vi "User Input block.vi"(7 "action":T1, 8 "error in":errorcluster, 10 "Pause!":bool) -> (0 "error out":errorcluster, 2 "Pause?":bool)   [LabVIEW 2018]
uses:
  type defines/Pause action.ctl
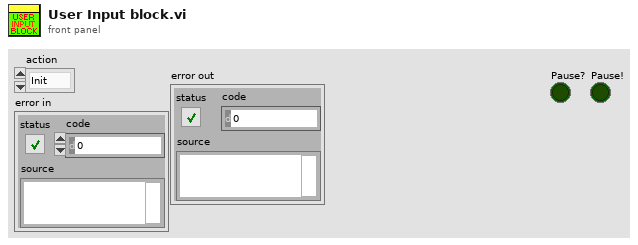
[diagram p1: front panel]
types:
  T1 = typedef "Pause action.ctl" = enum16{"Init", "get", "set"}
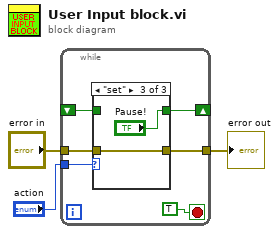
[diagram p0: block diagram]
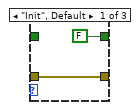
[diagram p2: hidden frame]
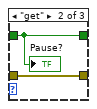
[diagram p3: hidden frame]
diagram:
  n1 = while {
    tunnel: "action" -> [w8]
    shift-right: [w7] -> _
    shift-left: _ -> [w6]
    tunnel: "error in" -> [w5]
    tunnel: [w4] -> w1
    stop <- TRUE stop-if-true
    n2 = case shown="\"set\"" w8 {
      tunnel: [FALSE w13 "Pause!"] -> w7
      tunnel: w6 -> [_ w13 _]
      tunnel: w5 -> [w10 w12 w14]
      tunnel: [w10 w12 w14] -> w4
      frame "Init", Default {
      }
      frame "get" {
        "Pause?" <- w13
      }
      frame "set" {
      }
    }
  }
  "error out" <- w1
